vi "Read Attributes.vi"(11 "Autotest_Result Msg":refnum<class "Autotest_Result Msg.lvclass">) -> (2 "Payload":cluster{"Autotest":bool, "Instr":string})   [LabVIEW 2020, in "Library Core.lvlib" / "Actor_Autotest.lvlib" / "Autotest_Result Msg.lvclass"]
uses:
  Autotest_Result Msg.lvclass
  Autotest_Result Msg.lvclass/Autotest_Result Msg.ctl
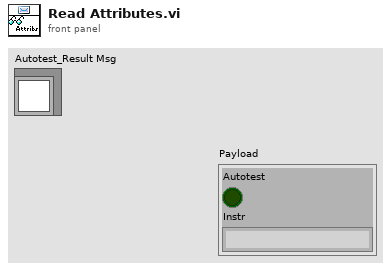
[diagram p1: front panel]
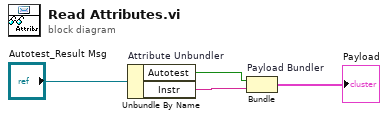
[diagram p0: block diagram]
diagram:
  n1 = Unbundle By Name "Attribute Unbundler"("Autotest_Result Msg") -> ("Autotest"=w2:bool, "Instr"=w1:string)
  n2 = Bundle "Payload Bundler"("Autotest"=w2, "Instr"=w1) -> (→"Payload":cluster{"Autotest":bool, "Instr":string})  [unwired: 1 in]
